vi "Read Discovery Service Key File.vi"(8 "error in (no error)":errorcluster, 11 "key file path":path) -> (0 "error out":errorcluster, 3 "key json":string)   [LabVIEW 2020, in "MeasurementLink Measurement Server.lvlib"]
uses:
  MeasurementLink Measurement Server.lvlib
  Error Strings Global.vi
  kernel32.dll
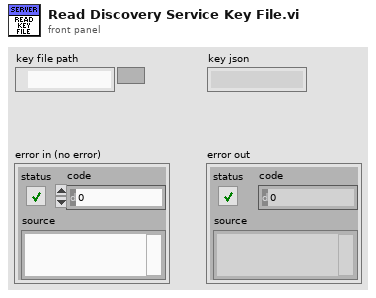
[diagram p1: front panel]
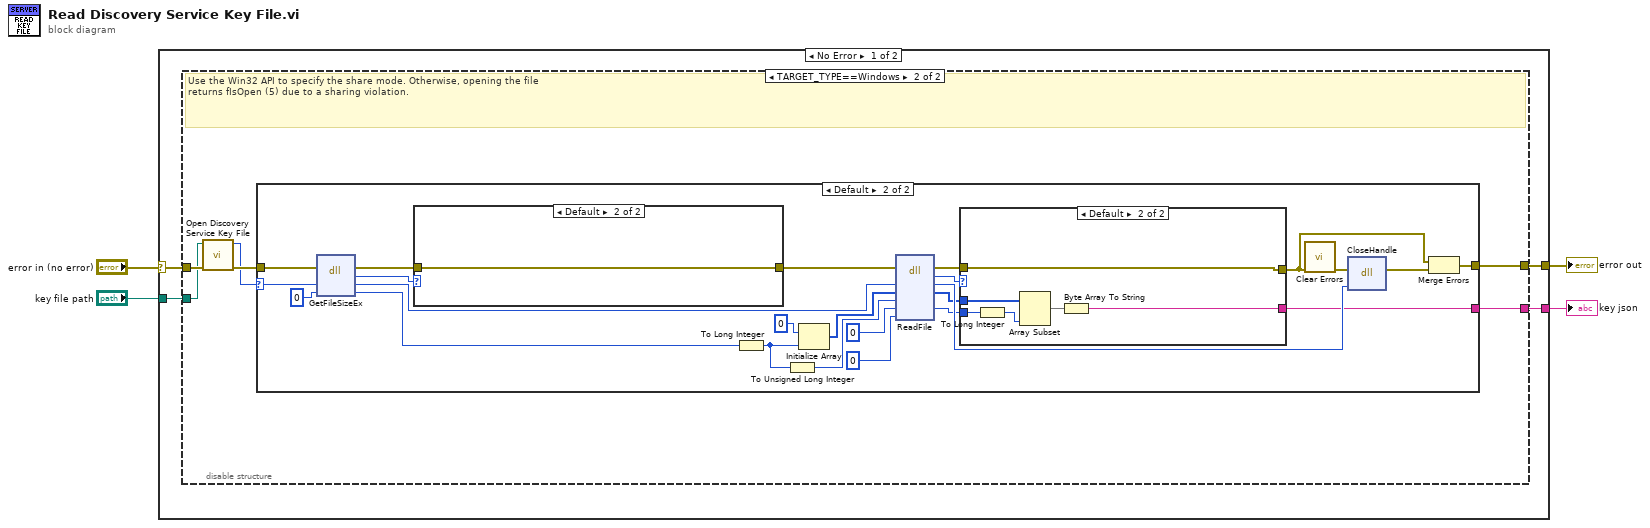
[diagram p0: block diagram]
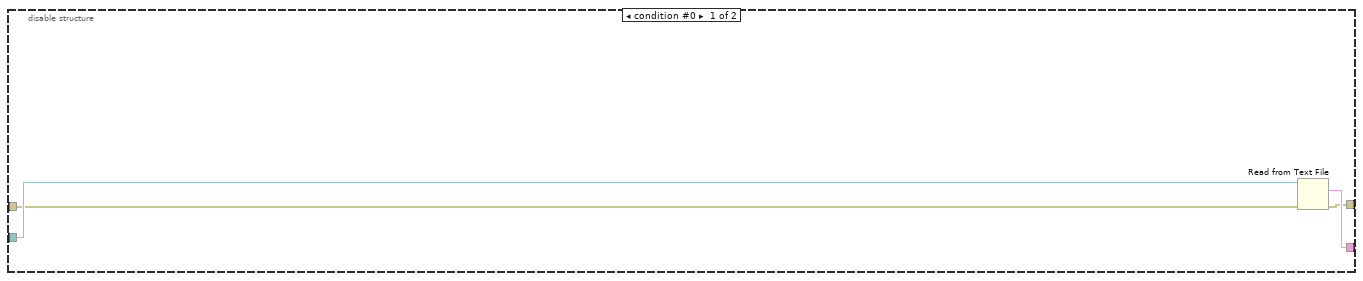
[diagram p2: hidden frame]
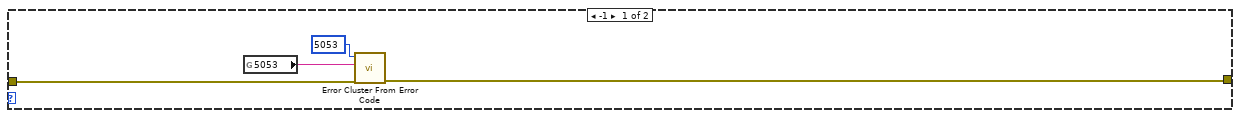
[diagram p3: hidden frame]
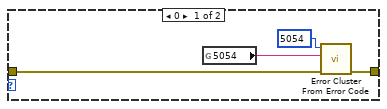
[diagram p4: hidden frame]
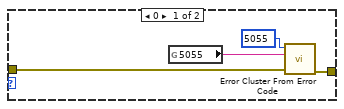
[diagram p5: hidden frame]
diagram:
  n1 = case shown="No Error" "error in (no error)" {
    selector: "error in (no error)" -> [w5 w62]
    tunnel: [w8 w62] -> w4
    tunnel: [w7 _] -> w3
    tunnel: "key file path" -> [w6 _]
    frame No Error {
      n2 = disable-structure shown="TARGET_TYPE==Windows" {
        disable-tunnel: w6 -> [w12 w15]
        disable-tunnel: w5 -> [w11 w16]
        disable-tunnel: [w10 w18] -> w7
        disable-tunnel: [w9 w17] -> w8
        frame condition #0 {
          n3 = Read from Text File(file (use dialog)=w12, error in=w11) -> (text=w10:string, error out=w9:errorcluster)  [unwired: 2 in, 2 out]
        }
        frame condition #1 (active) {
          # "Use the Win32 API to specify the share mode. Otherwise, opening the file\nreturns fIsOpen (5) due to a sharing violation."
          n4 = call "Open Discovery Service Key File.vi"("error in (no error)"=w16, "Key File"=w15) -> ("error out"=w14:errorcluster, "File Handle"=w13:i64)  [unwired: 8 in]
          n5 = case shown="Default" w13 {
            selector: w13 -> [_ w31]
            tunnel: w14 -> [w21 w29]
            tunnel: [w20 w40] -> w17
            tunnel: [_ w34] -> w18
            frame -1 {
              n6 = global read "Error Strings Global.vi" "5053"() -> (w19:string)
              n7 = call <vilib>:"Error Cluster From Error Code.vi"("error in (no error)"=w21, "error message (\"\")"=w19, "error code (0)"=5053) -> ("error out"=w20:errorcluster)  [unwired: 6 in]
            }
            frame Default {
              n8 = dll-call lib="kernel32.dll" fn="GetFileSizeEx"(error in=w29, "hFile"=w31, "lpFileSize"=i64 0) -> (error out=w26:errorcluster, "return type"=w25:i32, "hFile"=w30:i64, "lpFileSize"=w27:i64)  [unwired: 2 in, 1 out]
              n9 = case shown="Default" w25 {
                tunnel: w26 -> [w49 w51]
                tunnel: [w48 w51] -> w24
                frame 0 {
                  n10 = global read "Error Strings Global.vi" "5054"() -> (w47:string)
                  n11 = call <vilib>:"Error Cluster From Error Code.vi"("error in (no error)"=w49, "error message (\"\")"=w47, "error code (0)"=5054) -> ("error out"=w48:errorcluster)  [unwired: 6 in]
                }
                frame Default {
                }
              }
              n12 = To Long Integer(number=w27) -> (32bit integer=w23:i32)
              n13 = To Unsigned Long Integer(number=w23) -> (unsigned 32bit integer=w45:u32)
              n14 = Initialize Array(u8 0, w23) -> (w44:u8[])
              n15 = dll-call lib="kernel32.dll" fn="ReadFile"(error in=w24, "hFile"=w30, "lpBuffer"=w44, "nNumberOfBytesToRead"=w45, "lpNumberOfBytesRead"=u32 0, "lpOverlapped"=i64 0) -> (error out=w37:errorcluster, "return type"=w38:i32, "hFile"=w39:i64, "lpBuffer"=w36:u8[], "lpNumberOfBytesRead"=w35:u32)  [unwired: 4 in, 1 out]
              n16 = case shown="Default" w38 {
                tunnel: w37 -> [w54 w57]
                tunnel: [w53 w57] -> w32
                tunnel: w36 -> [_ w61]
                tunnel: w35 -> [_ w60]
                tunnel: [_ w56] -> w34
                frame 0 {
                  n17 = global read "Error Strings Global.vi" "5055"() -> (w52:string)
                  n18 = call <vilib>:"Error Cluster From Error Code.vi"("error in (no error)"=w54, "error message (\"\")"=w52, "error code (0)"=5055) -> ("error out"=w53:errorcluster)  [unwired: 6 in]
                }
                frame Default {
                  n19 = To Long Integer(number=w60) -> (32bit integer=w59:i32)
                  n20 = Array Subset(array=w61, length=w59) -> (w58:u8[])  [unwired: 1 in]
                  n21 = Byte Array To String(unsigned byte array=w58) -> (string=w56:string)
                }
              }
              n22 = call <vilib>:"Clear Errors.vi"("error in (no error)"=w32) -> ("error out"=w33:errorcluster)  [unwired: 5 in, 1 out]
              n23 = dll-call lib="kernel32.dll" fn="CloseHandle"(error in=w33, "hObject"=w39) -> (error out=w41:errorcluster)  [unwired: 4 in, 1 out]
              n24 = Merge Errors(w32, w41) -> (w40:errorcluster)
            }
          }
        }
      }
    }
    frame Error {
    }
  }
  "error out" <- w4
  "key json" <- w3
